vi "Write Address 2.vi"(8 "error in (no error)":errorcluster, 10 "Address":string="DEV3523", 11 "ZI Lockin in":refnum<class "ZI Lockin.lvclass">) -> (0 "error out":errorcluster, 3 "ZI Lockin out":refnum<class "ZI Lockin.lvclass">)   [LabVIEW 2017]
uses:
  ZI Lockin.lvclass
  C:/github/NHMFL_Core/Libraries/Instruments/Simple VISA Reader/Simple VISA Reader Driver.lvclass
  C:/github/NHMFL_Core/Libraries/Instruments/VISA Instrument/VISA Instrument.lvclass
  C:/github/NHMFL_Core/Libraries/Instruments/Instrument Driver/Instrument Driver.lvclass
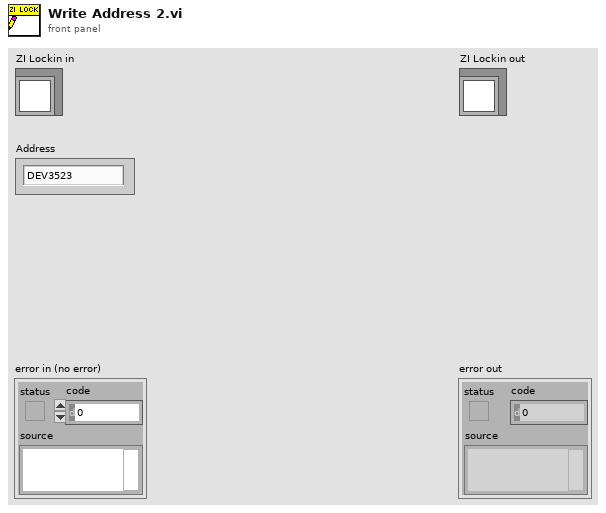
[diagram p1: front panel]
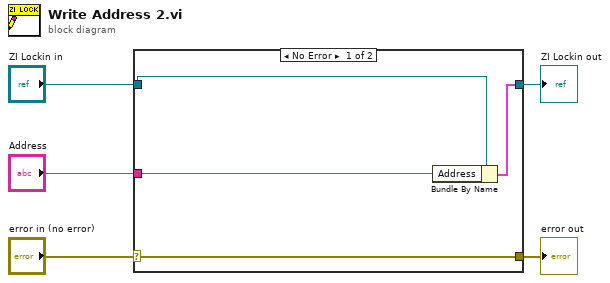
[diagram p0: block diagram]
diagram:
  n1 = case shown="No Error" "error in (no error)" {
    selector: "error in (no error)" -> [w9 w10]
    tunnel: [w9 w10] -> w4
    tunnel: [w7 w11] -> w2
    tunnel: "ZI Lockin in" -> [w8 w11]
    tunnel: "Address" -> [w6 _]
    frame No Error {
      n2 = Bundle By Name(cluster=w8, "Address"=w6) -> (w7:cluster{})
    }
    frame Error {
    }
  }
  "error out" <- w4
  "ZI Lockin out" <- w2
